vi "ILA_NO.vi"() -> ()   [LabVIEW 2017]
panel:
  out "floor(x/y)":u8=3
  in  "ILA channel":u8=27
  out "Out":u8=27 format="%.0x"
  in  "address":string="10.3.173.20"
  in  "error in (no error)":errorcluster
  out "error out":errorcluster
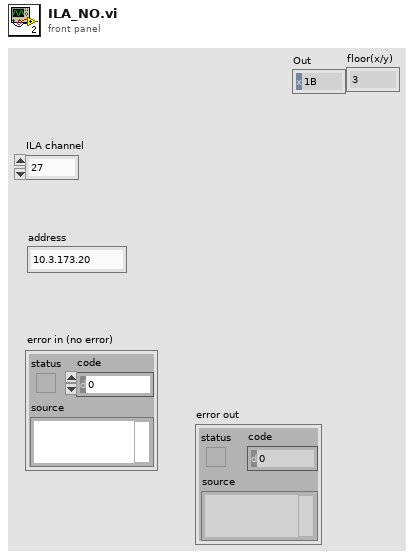
[diagram p1: front panel]
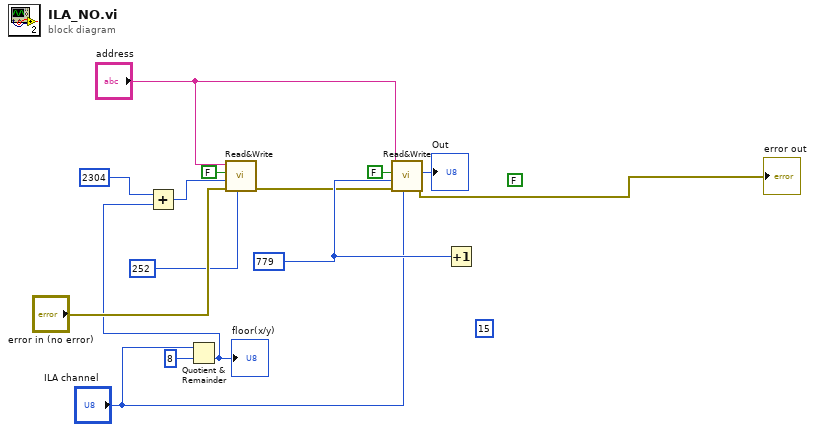
[diagram p0: block diagram]
diagram:
  (unwired) FALSE ("Read (TRUE)")
  (unwired) u8 15 ("In")
  w13 = u32 779 ("Address")
  n1 = Quotient & Remainder(x="ILA channel", y=u8 8) -> (floor(x/y)=w3:u8)  [unwired: 1 out]
  "floor(x/y)" <- w3
  n2 = Add(x=u32 2304 ("Address"), y=w3) -> (x+y=w1:u32)
  n3 = call "Read&Write.vi"("In"=u32 252 ("Address"), "error in (no error)"="error in (no error)", "Address"=w1, "Read (TRUE)"=FALSE, "address"="address") -> ("error out"=w8:errorcluster)  [unwired: 5 in, 1 out]
  n4 = call "Read&Write.vi"("In"="ILA channel", "error in (no error)"=w8, "Address"=w13, "Read (TRUE)"=FALSE, "address"="address") -> ("error out"=→"error out":errorcluster, "Out"=→"Out":u8)  [unwired: 5 in]
  n5 = Increment(x=w13) -> ()  [unwired: 1 out]
